vi "Send.vi"(7 "Message Priority (Normal)":T1=enum."Normal", 8 "error in (no error)":errorcluster, 9 "Message":refnum<class "Message.lvclass">, 10 "Actor in":refnum<class "Actor.lvclass">, 11 "Targetted Msg in":refnum<class "Targetted Msg.lvclass">) -> (0 "error out":errorcluster, 1 "Dropped?":bool, 2 "Actor out":refnum<class "Actor.lvclass">)   [LabVIEW 2020, in "Publisher.lvlib" / "Targetted Msg.lvclass"]
doc: "Send a Message somewhere through the Publisher. \nThe default implementation has no targetting so instead of sending the Sender Msg the Message is sent in a Publish Msg."
uses:
  Targetted Msg.lvclass
  C:/Current projects/WS/Framework/Framework/Actors/Publisher/Publisher Messages/Sender Msg/Sender Msg.lvclass
  C:/Current projects/WS/Framework/Framework/Actors/Publisher/Publisher Messages/Publisher Msg/Publisher Msg.lvclass
  PPL/HDH.Actor Framework.Core.Actor.lvlibp/1abvi3w/vi.lib/ActorFramework/Message Enqueuer/Message Priority.ctl
  PPL/HDH.Actor Framework.Core.Actor.lvlibp/1abvi3w/vi.lib/ActorFramework/Message/Message.lvclass
  PPL/HDH.Actor Framework.Core.Actor.lvlibp/1abvi3w/vi.lib/ActorFramework/Actor/Actor.lvclass
  Targetted Msg.lvclass/Targetted Msg.ctl
  Sender Msg/Sender Msg.lvclass/Sender Msg.ctl
  Publisher Msg/Publisher Msg.lvclass
  Sender Msg/Sender Msg.lvclass
  PPL/HDH.Actor Framework.Core.Actor.lvlibp/1abvi3w/vi.lib/ActorFramework/Message Enqueuer/Message Enqueuer.lvclass
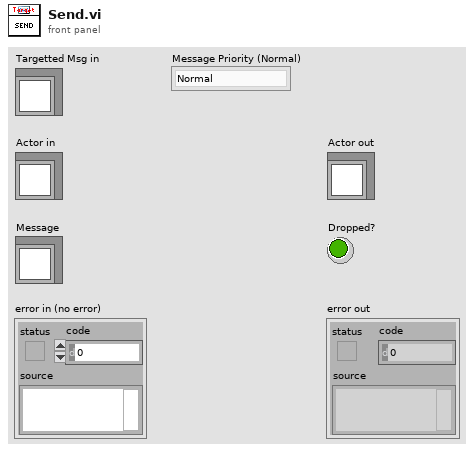
[diagram p1: front panel]
types:
  T1 = typedef "HDH.Actor Framework.Core.Actor.lvlibp/Message Enqueuer.lvclass/Message Priority.ctl" = enum16{"Low", "Normal", "High"}
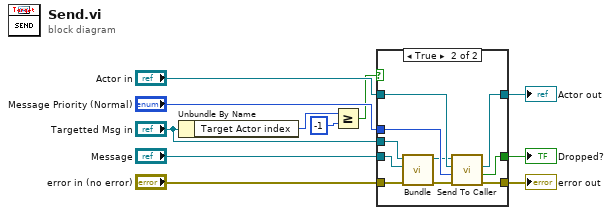
[diagram p0: block diagram]
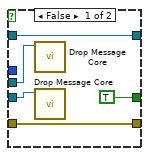
[diagram p2: hidden frame]
diagram:
  n1 = Unbundle By Name("Targetted Msg in") -> ("Target Actor index"=w3:i32)
  n2 = Greater Or Equal?(x=w3, y=-1) -> (x >= y?=w1:bool)
  n3 = case shown="True" w1 {
    tunnel: "Message Priority (Normal)" -> [_ w26]
    tunnel: "Actor in" -> [w16 w25]
    tunnel: [w16 w24] -> w9
    tunnel: "Message" -> [w14 w23]
    tunnel: "error in (no error)" -> [w12 w22]
    tunnel: [TRUE ("Msg Dropped?") w19] -> w6
    tunnel: [w12 w18] -> w5
    tunnel: "Targetted Msg in" -> [w15 w17]
    frame False {
      n4 = call-dynamic "Drop Message Core.vi"("Message in"=w15) -> ()  [unwired: 11 in]
      n5 = call-dynamic "Drop Message Core.vi"("Message in"=w14) -> ()  [unwired: 11 in]
    }
    frame True {
      n6 = call "Bundle.vi"("error in (no error)"=w22, "Message"=w23, "Targetted Msg in"=w17) -> ("error out"=w20:errorcluster, "Targetted Msg out"=w21:refnum<class "Targetted Msg.lvclass">)  [unwired: 7 in]
      n7 = call "Send To Caller.vi"("error in (no error)"=w20, "Message Priority (Normal)"=w26, "Actor in"=w25, "Publisher Msg in"=w21) -> ("error out"=w18:errorcluster, "Msg Dropped?"=w19:bool, "Actor out"=w24:refnum<class "Actor.lvclass">)  [unwired: 5 in]
    }
  }
  "error out" <- w5
  "Actor out" <- w9
  "Dropped?" <- w6
